vi "SPD.HV_Grid Initial Range Search Controller.vi"(0 "HV_bias":dbl, 1 "state":T2, 2 "DCRRange":T3, 5 "HV_GridParams":T1, 9 "DCR":dbl, 11 "Error In":errorcluster) -> (3 "next state":T2, 4 "HV_bias Next":dbl, 6 "HV_bias max":dbl, 8 "HV_bias min":dbl, 10 "done":bool, 15 "Error Out":errorcluster)   [LabVIEW 2018]
uses:
  SubVIs/Min_Max.ctl
  HV_Grid Range Search States.ctl
  SPD.HV_Grid Test Params.ctl
  SubVIs/comparison mode.ctl
  <vilib>/Utility/error.llb/Error Cluster From Error Code.vi
  <vilib>/ErrorRing/Error Ring.xnode
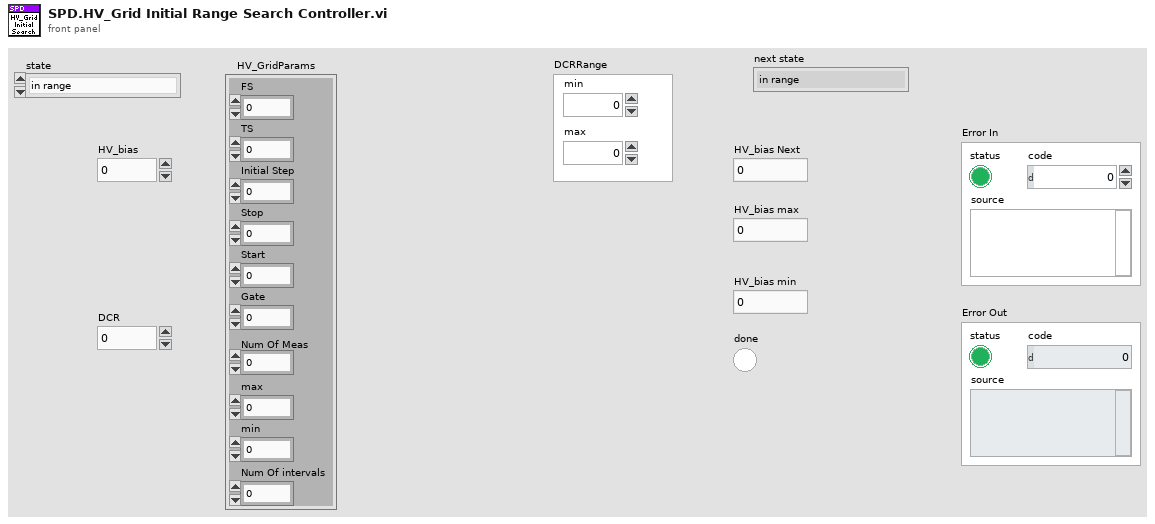
[diagram p1: front panel]
types:
  T1 = typedef "SPD.HV_Grid Test Params.ctl" = cluster{"FS":i32, "TS":i32, "Initial Step":dbl, "Stop":dbl, "Start":dbl, "Gate":dbl, "Num Of Meas":i32, "max":dbl, "min":dbl, "Num Of intervals":i32}
  T2 = typedef "HV_Grid Range Search States.ctl" = enum16{"in range", "max", "min"}
  T3 = typedef "Min_Max.ctl" = cluster{"min":dbl, "max":dbl}
  T4 = typedef "comparison mode.ctl" = enum16{"in range", "bigger then min", "bigger then max", "less then min", "less then max"}
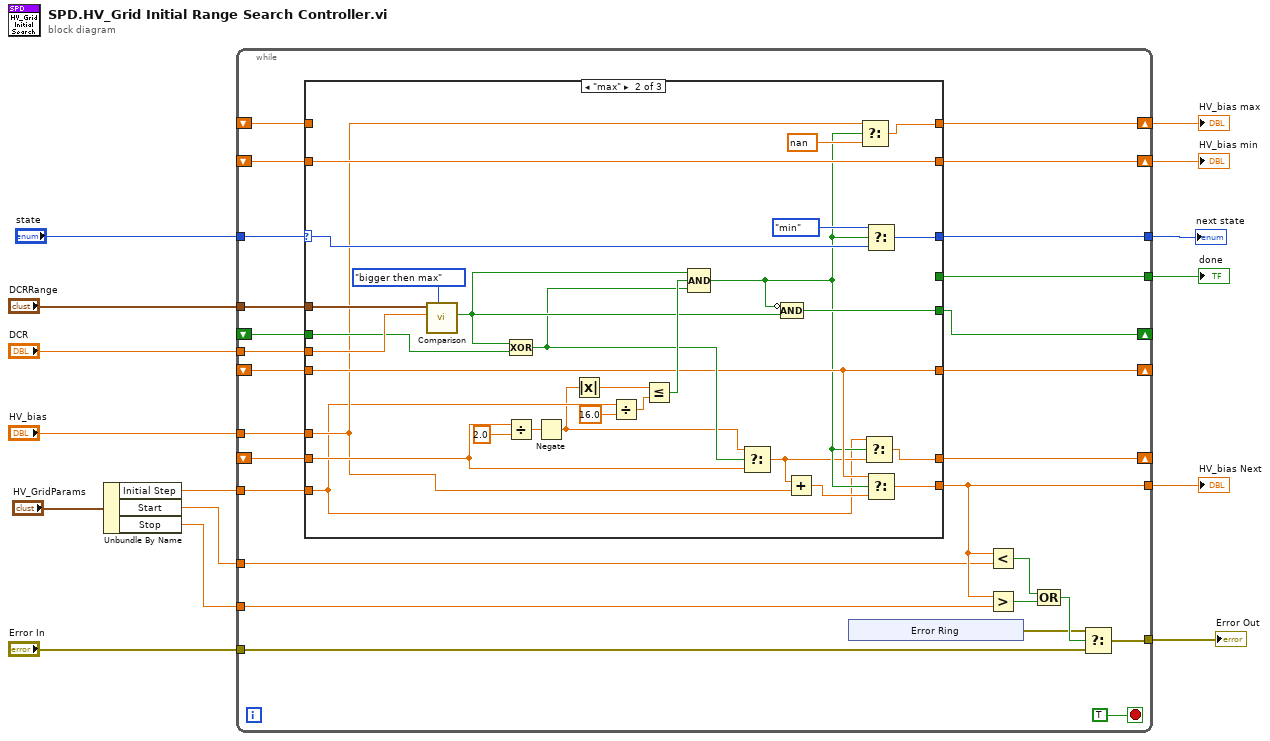
[diagram p0: block diagram]
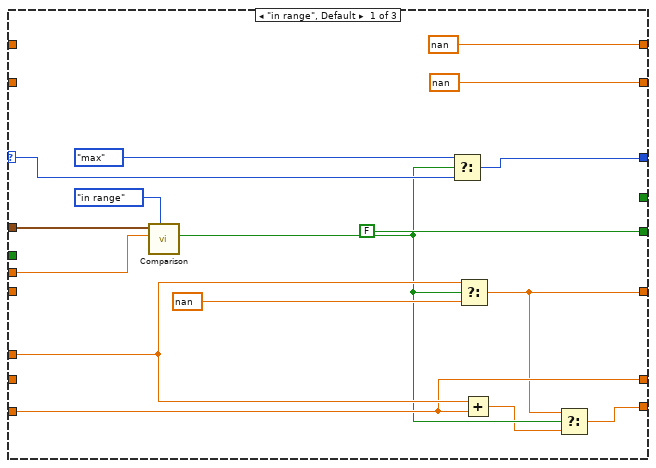
[diagram p2: hidden frame]
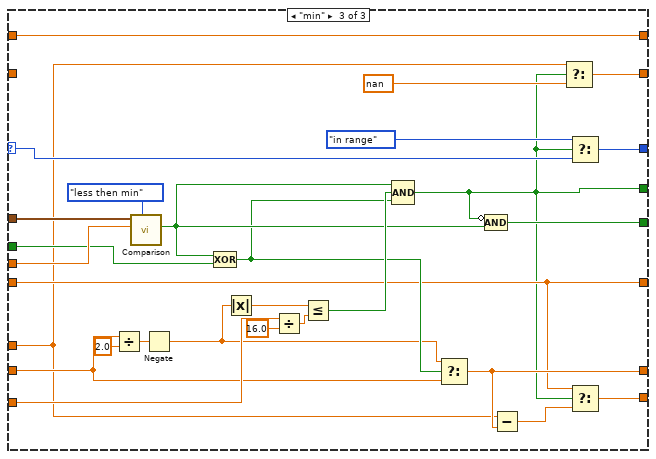
[diagram p3: hidden frame]
diagram:
  n1 = Unbundle By Name("HV_GridParams") -> ("Initial Step"=w3:dbl, "Start"=w2:dbl, "Stop"=w1:dbl)
  n2 = while {
    tunnel: "DCR" -> [w39]
    shift-right: [w28] -> w13
    shift-left: _ -> [w27]
    shift-right: [w29] -> w12
    shift-left: _ -> [w26]
    tunnel: "DCRRange" -> [w40]
    tunnel: "HV_bias" -> [w36]
    shift-right: [w37] -> _
    shift-left: _ -> [w35]
    tunnel: w3 -> [w34]
    tunnel: [w24] -> w10
    shift-right: [w33] -> _
    shift-left: _ -> [w32]
    shift-right: [w31] -> _
    shift-left: _ -> [w30]
    tunnel: [w25] -> w9
    tunnel: w2 -> [w23]
    tunnel: w1 -> [w22]
    tunnel: "Error In" -> [w18]
    tunnel: [w17] -> w7
    tunnel: "state" -> [w41]
    tunnel: [w38] -> w5
    stop <- TRUE stop-if-true
    n3 = case shown="\"max\"" w41 {
      selector: w41 -> [w52 w87 w114]
      tunnel: w40 -> [w58 w91 w119]
      tunnel: w39 -> [w62 w90 w118]
      tunnel: [w60 w85 w112] -> w38
      tunnel: [w51 w73 w99] -> w37
      tunnel: w36 -> [w57 w71 w98]
      tunnel: w35 -> [_ w73 w99]
      tunnel: w34 -> [w56 w65 w117]
      tunnel: [w48 w74 w100] -> w24
      tunnel: [w56 w68 w103] -> w33
      tunnel: w32 -> [_ w77 w104]
      tunnel: [FALSE ("result") w76 w102] -> w31
      tunnel: w30 -> [_ w82 w109]
      tunnel: [nan ("element") w72 w95] -> w29
      tunnel: [nan ("element") w70 w94] -> w28
      tunnel: w27 -> [_ _ w94]
      tunnel: w26 -> [_ w72 _]
      tunnel: [_ _ w96] -> w25
      frame "in range", Default {
        n4 = call "Comparison.vi"("Comparison Mode"=comparison_mode."in range", "value"=w62, "minMax"=w58) -> ("result"=w50:bool)  [unwired: 8 in]
        n5 = Select(t=HV_Grid_Range_Search_States."max" ("HV_Grid Range Search States"), s=w50, f=w52) -> (s? t:f=w60:T2)
        n6 = Select(t=w57, s=w50, f=nan ("element")) -> (s? t:f=w51:dbl)
        n7 = Add(x=w57, y=w56) -> (x+y=w49:dbl)
        n8 = Select(t=w51, s=w50, f=w49) -> (s? t:f=w48:dbl)
      }
      frame "max" {
        n9 = call "Comparison.vi"("Comparison Mode"=comparison_mode."bigger then max", "value"=w90, "minMax"=w91) -> ("result"=w83:bool)  [unwired: 8 in]
        n10 = Divide(x=w77, y=2.0) -> (x/y=w79:dbl)
        n11 = Compound Arithmetic op=XOR(w83, w82) -> (w78:bool)
        n12 = Negate(x=w79) -> (-x=w64:dbl)
        n13 = Absolute Value(x=w64) -> (abs(x)=w81:dbl)
        n14 = Divide(x=w65, y=16.0) -> (x/y=w88:dbl)
        n15 = Less Or Equal?(x=w81, y=w88) -> (x <= y?=w84:bool)
        n16 = Compound Arithmetic op=AND(w83, w84, w78) -> (w67:bool)
        n17 = Select(t=w64, s=w78, f=w77) -> (s? t:f=w66:dbl)
        n18 = Compound Arithmetic op=AND(invert w67, w83) -> (w76:bool)
        n19 = Add(x=w66, y=w71) -> (x+y=w75:dbl)
        n20 = Select(t=w71, s=w67, f=nan) -> (s? t:f=w70:dbl)
        n21 = Select(t=w65, s=w67, f=w66) -> (s? t:f=w68:dbl)
        n22 = Select(t=HV_Grid_Range_Search_States."min", s=w67, f=w87) -> (s? t:f=w85:T2)
        n23 = Select(t=w73, s=w67, f=w75) -> (s? t:f=w74:dbl)
      }
      frame "min" {
        n24 = Divide(x=w104, y=2.0) -> (x/y=w106:dbl)
        n25 = call "Comparison.vi"("Comparison Mode"=comparison_mode."less then min", "value"=w118, "minMax"=w119) -> ("result"=w110:bool)  [unwired: 8 in]
        n26 = Negate(x=w106) -> (-x=w93:dbl)
        n27 = Compound Arithmetic op=XOR(w110, w109) -> (w105:bool)
        n28 = Absolute Value(x=w93) -> (abs(x)=w108:dbl)
        n29 = Divide(x=w117, y=16.0) -> (x/y=w115:dbl)
        n30 = Less Or Equal?(x=w108, y=w115) -> (x <= y?=w111:bool)
        n31 = Compound Arithmetic op=AND(w110, w111, w105) -> (w96:bool)
        n32 = Select(t=w93, s=w105, f=w104) -> (s? t:f=w103:dbl)
        n33 = Compound Arithmetic op=AND(invert w96, w110) -> (w102:bool)
        n34 = Subtract(x=w98, y=w103) -> (x-y=w101:dbl)
        n35 = Select(t=w98, s=w96, f=nan) -> (s? t:f=w95:dbl)
        n36 = Select(t=HV_Grid_Range_Search_States."in range", s=w96, f=w114) -> (s? t:f=w112:T2)
        n37 = Select(t=w99, s=w96, f=w101) -> (s? t:f=w100:dbl)
      }
    }
    n38 = xnode "Error Ring"() -> ("error out"=w16:errorcluster)
    n39 = Less?(x=w24, y=w23) -> (x < y?=w21:bool)
    n40 = Greater?(x=w24, y=w22) -> (0:w20:bool)
    n41 = Compound Arithmetic op=OR(w21, w20) -> (w19:bool)
    n42 = Select(t=w16, s=w19, f=w18) -> (s? t:f=w17:errorcluster)
  }
  "done" <- w9
  "HV_bias min" <- w12
  "HV_bias max" <- w13
  "HV_bias Next" <- w10
  "Error Out" <- w7
  "next state" <- w5
